vi "Main Page.vi"(8 "error in (no error)":errorcluster, 11 "Node Ptr":T2 format="%.0x") -> (0 "error out":errorcluster)   [LabVIEW 2010]
uses:
  <vilib>/NI Veristand/Custom Device API/Custom Device API.lvlib
  <vilib>/NI VeriStand/Custom Device API/Set Item Property (Variant).vi
  <vilib>/NI VeriStand/Custom Device API/Get Item Property (Variant).vi
  <vilib>/NI VeriStand/Custom Device API/Custom Device Item Ref.ctl
  Configuration Data.ctl
panel:
  in  "Decimation":i32=1
  in  "Description":string
  in  "Name":string
  in  "Configuration Data":T1
  in  "Header":cluster{"Section Name":string}={"Section Name"="Custom Device Item Settings"}
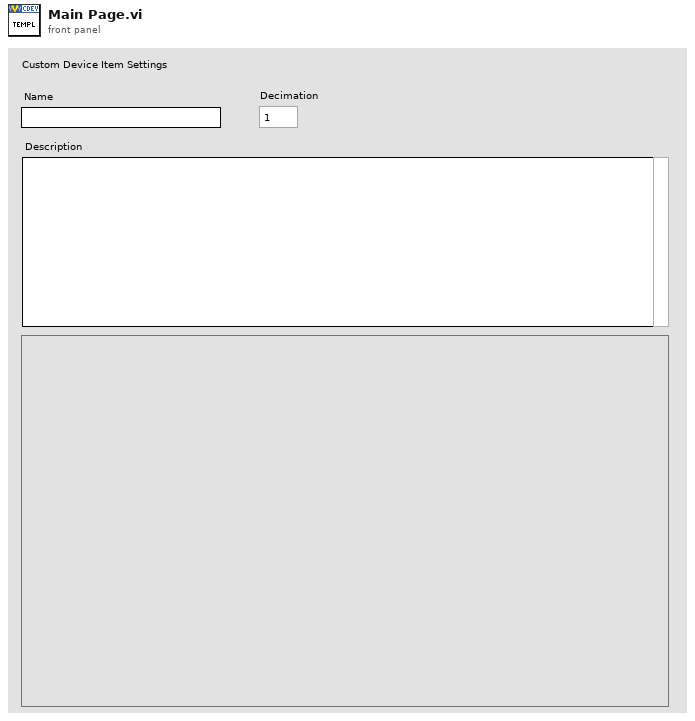
[diagram p1: front panel]
types:
  T1 = typedef "Configuration Data.ctl" = cluster{}
  T2 = typedef "Custom Device API.lvlib/Custom Device Item Ref.ctl" = u64
  T3 = typedef "Custom Device API.lvlib/Custom Device Item Info.ctl" = cluster{"Name":string, "Is Channel":bool, "GUID":string}
  T4 = typedef "Custom Device API.lvlib/Custom Device Commands.ctl" = enum16{"Default", "Item renamed", "Shutdown", "Dynamic button pressed"}
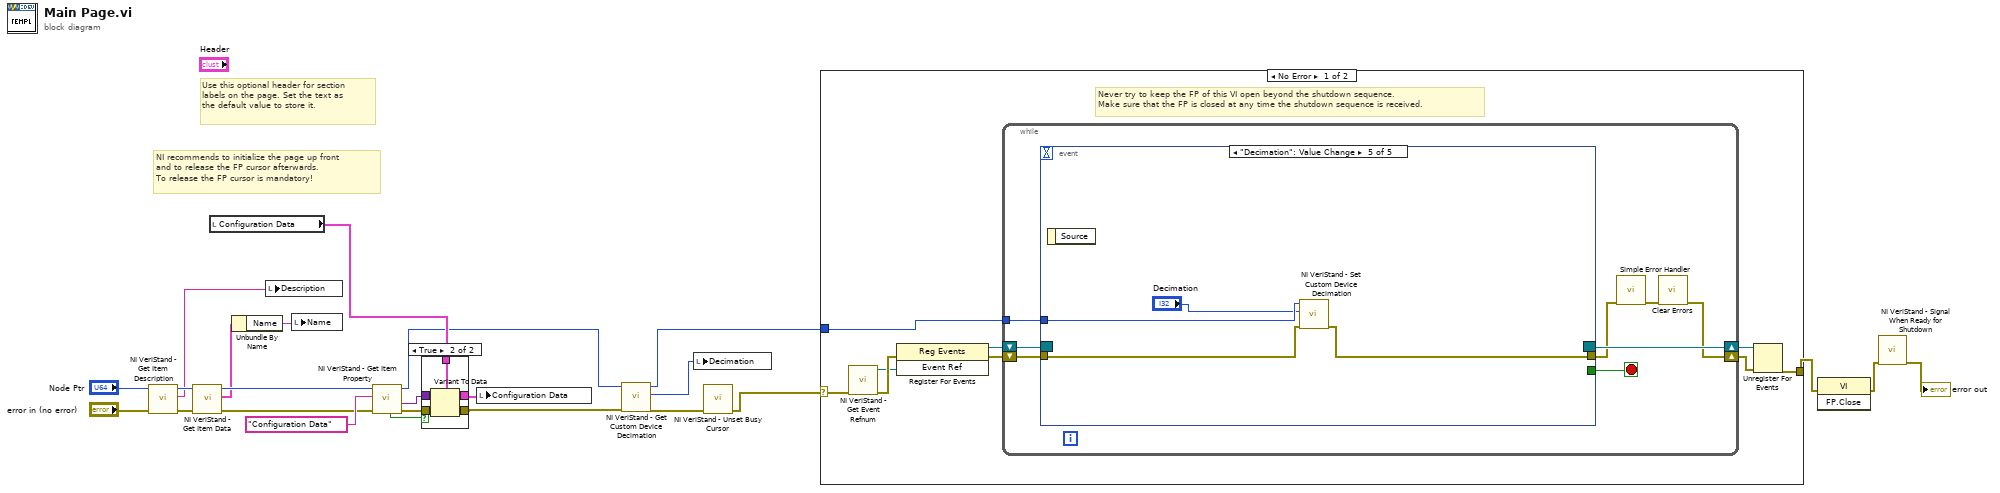
[diagram p0: block diagram]
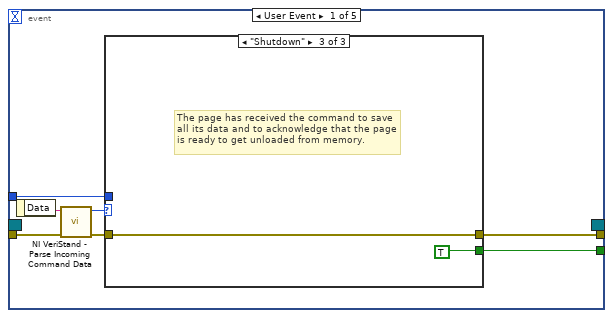
[diagram p3: hidden frame]
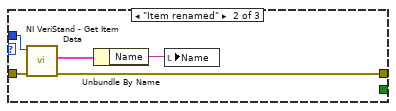
[diagram p5: hidden frame]
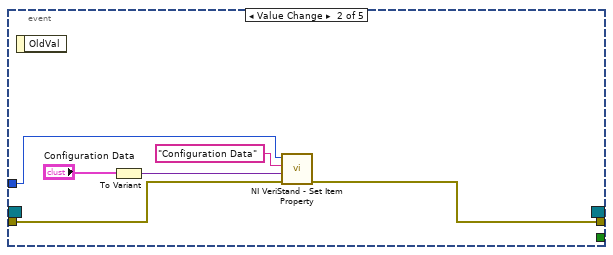
[diagram p6: hidden frame]
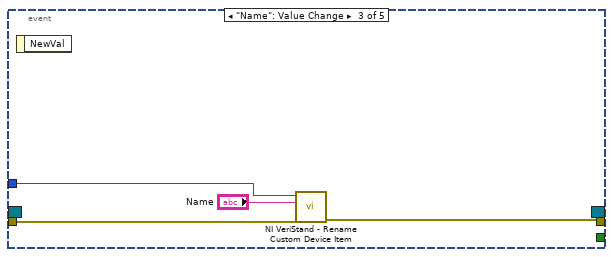
[diagram p7: hidden frame]
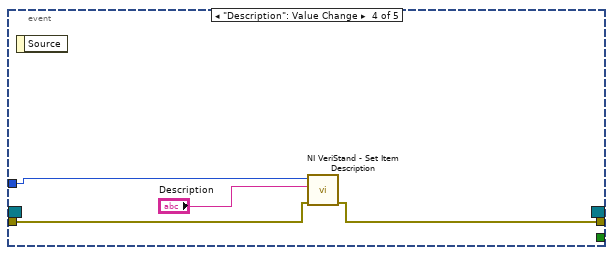
[diagram p8: hidden frame]
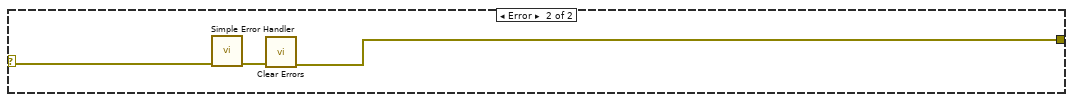
[diagram p9: hidden frame]
diagram:
  # "Use this optional header for section labels on the page. Set the text as the default value to store it."
  # "NI recommends to initialize the page up front\nand to release the FP cursor afterwards.\nTo release the FP cursor is mandatory!"
  n1 = call <vilib>:"NI VeriStand - Get Item Description.vi"("error in (no error)"="error in (no error)", "Item Ref in"="Node Ptr") -> ("error out"=w16:errorcluster, "Description"=w6:string, "Item Ref out"=w17:T2)  [unwired: 7 out]
  n2 = call <vilib>:"NI VeriStand - Get Item Data.vi"("error in (no error)"=w16, "Item Ref in"=w17) -> ("error out"=w13:errorcluster, "Item Info"=w9:T3, "Item Ref out"=w15:T2)  [unwired: 7 out]
  n3 = local read "Configuration Data"() -> (w18:T1)
  n4 = Unbundle By Name(w9) -> ("Name"=w7:string)
  n5 = local write "Description"(w6) -> ()
  n6 = local write "Name"(w7) -> ()
  n7 = call-poly <vilib>:"NI VeriStand - Get Item Property.vi"("error in (no error)"=w13, "Property Name"="Configuration Data", "Item Ref in"=w15) -> ("error out"=w12:errorcluster, "Value"=w11:variant, "Item Ref out"=w4:T2, "Found?"=w8:bool)  [unwired: 5 in]
  n8 = case shown="True" w8 {
    tunnel: w12 -> [w25 w31]
    tunnel: w11 -> [_ w30]
    tunnel: [w26 w29] -> w10
    tunnel: [w25 w28] -> w5
    tunnel: w18 -> [w26 w27]
    frame False {
    }
    frame True {
      n9 = Variant To Data(error in=w31, Variant=w30, type=w27) -> (error out=w28:errorcluster, data=w29:T1)
    }
  }
  n10 = local write "Configuration Data"(w10) -> ()
  n11 = call <vilib>:"NI VeriStand - Get Custom Device Decimation.vi"("error in (no error)"=w5, "Device Ref in"=w4) -> ("error out"=w2:errorcluster, "Decimation"=w1:i32, "Device Ref out"=w3:T2)  [unwired: 7 in]
  n12 = local write "Decimation"(w1) -> ()
  n13 = call <vilib>:"NI VeriStand - Unset Busy Cursor.vi"("error in (no error)"=w2) -> ("error out"=w20:errorcluster)  [unwired: 10 out]
  n14 = case shown="No Error" w20 {
    selector: w20 -> [w33 w84]
    tunnel: [w37 w82] -> w24
    tunnel: w3 -> [w32 _]
    frame No Error {
      # "Never try to keep the FP of this VI open beyond the shutdown sequence.\nMake sure that the FP is closed at any time the shutdown sequence is received."
      n15 = call <vilib>:"NI VeriStand - Get Event Refnum.vi"("error in (no error)"=w33) -> ("error out"=w40:errorcluster, "Event Ref"=w36:refnum<user-event>)  [unwired: 9 out]
      n16 = register-events(error in=w40, w36) -> (reference out=w34:refnum<event-registration>, error out=w35:errorcluster)  [unwired: 1 in]
      n17 = while {
        shift-right: [w42] -> w38
        shift-left: w35 -> [w47]
        shift-right: [w48] -> w39
        shift-left: w34 -> [w46]
        tunnel: w32 -> [w41]
        stop <- w45 stop-if-true
        n18 = event shown="[4] \"Decimation\": Value Change" {
          selector: w46 -> [_ _ _ _ _]
          dyn-events: [_ _ _ _ _] -> w48
          timeout: _ -> [_ _ _ _ _]
          tunnel: w47 -> [w55 w66 w71 w76 w79]
          tunnel: [w51 _ _ _ _] -> w45
          tunnel: [w50 w65 w70 w74 w78] -> w44
          tunnel: w41 -> [w49 w67 w72 w77 w81]
          event User Event {
            n19 = event-data() -> ("Data"=w54:string)  [unwired: 1 out]
            n20 = call <vilib>:"NI VeriStand - Parse Incoming Command Data.vi"("error in (no error)"=w55, "Data"=w54) -> ("error out"=w53:errorcluster, "Action"=w52:T4)  [unwired: 8 out]
            n21 = case shown="\"Shutdown\"" w52 {
              tunnel: w53 -> [w56 w61 w62]
              tunnel: [_ _ TRUE] -> w51
              tunnel: [w56 w59 w62] -> w50
              tunnel: w49 -> [_ w58 _]
              frame "Default", Default {
              }
              frame "Item renamed" {
                n22 = call <vilib>:"NI VeriStand - Get Item Data.vi"("error in (no error)"=w61, "Item Ref in"=w58) -> ("error out"=w59:errorcluster, "Item Info"=w60:T3)  [unwired: 8 out]
                n23 = Unbundle By Name(w60) -> ("Name"=w57:string)
                n24 = local write "Name"(w57) -> ()
              }
              frame "Shutdown" {
                # "The page has received the command to save all its data and to acknowledge that the page is ready to get unloaded from memory."
              }
            }
          }
          event Value Change {
            n25 = event-data() -> ()  [unwired: 2 out]
            n26 = To Variant(anything="Configuration Data") -> (Variant=w69:variant)
            n27 = call-poly <vilib>:"NI VeriStand - Set Item Property.vi"("error in (no error)"=w66, "Value"=w69, "Property Name"="Configuration Data", "Item Ref in"=w67) -> ("error out"=w65:errorcluster)  [unwired: 5 in, 2 out]
          }
          event "Name": Value Change {
            n28 = event-data() -> ()  [unwired: 2 out]
            n29 = call <vilib>:"NI VeriStand - Rename Custom Device Item.vi"("error in (no error)"=w71, "New Name"="Name", "Item Ref in"=w72) -> ("error out"=w70:errorcluster)  [unwired: 8 out]
          }
          event "Description": Value Change {
            n30 = event-data() -> ()  [unwired: 2 out]
            n31 = call <vilib>:"NI VeriStand - Set Item Description.vi"("error in (no error)"=w76, "Description"="Description", "Item Ref in"=w77) -> ("error out"=w74:errorcluster)  [unwired: 8 out]
          }
          event "Decimation": Value Change {
            n32 = event-data() -> ()  [unwired: 2 out]
            n33 = call <vilib>:"NI VeriStand - Set Custom Device Decimation.vi"("error in (no error)"=w79, "Decimation"="Decimation", "Device Ref in"=w81) -> ("error out"=w78:errorcluster)  [unwired: 7 in, 1 out]
          }
        }
        n34 = call <vilib>:"Simple Error Handler.vi"("error in (no error)"=w44) -> ("error out"=w43:errorcluster)  [unwired: 1 in, 7 out]
        n35 = call <vilib>:"Clear Errors.vi"("error in (no error)"=w43) -> ("error out"=w42:errorcluster)  [unwired: 6 out]
      }
      n36 = Unregister For Events(event registration refnum=w39, error in=w38) -> (error out=w37:errorcluster)
    }
    frame Error {
      n37 = call <vilib>:"Simple Error Handler.vi"("error in (no error)"=w84) -> ("error out"=w83:errorcluster)  [unwired: 1 in, 7 out]
      n38 = call <vilib>:"Clear Errors.vi"("error in (no error)"=w83) -> ("error out"=w82:errorcluster)  [unwired: 6 out]
    }
  }
  n39 = invoke class="VI" method="FP.Close"(error in=w24) -> (error out=w23:errorcluster)  [unwired: 2 in, 2 out]
  n40 = call <vilib>:"NI VeriStand - Signal When Ready for Shutdown.vi"("error in (no error)"=w23) -> ("error out"=→"error out":errorcluster)  [unwired: 10 out]
